vi "Init Tree.vi"(8 "error in":errorcluster) -> (0 "error out":errorcluster, 3 "Tree Map out":refnum<class "Project Tree Map.lvclass">)   [LabVIEW 2020, in "VI Properties Editor.lvlib" / "Project Tree Map.lvclass"]
doc: "Initializes the tree."
uses:
  Project Tree Map.lvclass
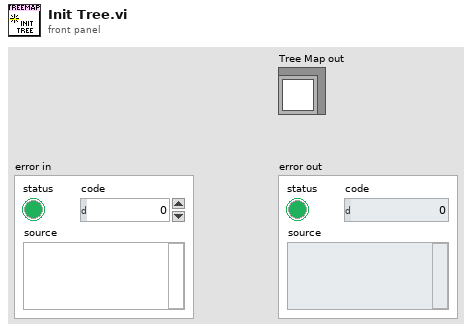
[diagram p1: front panel]
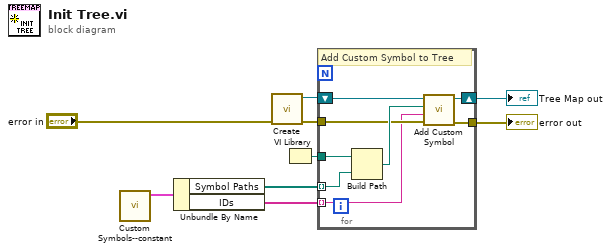
[diagram p0: block diagram]
diagram:
  n1 = call "Custom Symbols--constant.vi"() -> ("Custom Symbols"=w4:cluster{"Symbol Paths":path[], "IDs":string[]})  [unwired: 11 in]
  n2 = Unbundle By Name(w4) -> ("Symbol Paths"=w3:path[], "IDs"=w2:string[])
  n3 = call "Create.vi"("error in (no error)"="error in") -> ("error out"=w5:errorcluster, "Tree Map out"=w1:refnum<class "Project Tree Map.lvclass">)  [unwired: 9 in]
  n4 = VI Library() -> (path=w9:path)
  n5 = for {
    tunnel: w9 -> [w17]
    shift-right: [w14] -> w6
    shift-left: w1 -> [w16]
    tunnel: w5 -> [w12]
    tunnel: [w13] -> w8
    tunnel: w2 -> [w10] mode=indexing
    tunnel: w3 -> [w11] mode=indexing
    # "Add Custom Symbol to Tree"
    n6 = Build Path(base path=w17, name or relative path=w11) -> (appended path=w15:path)
    n7 = call "Add Custom Symbol.vi"("error in"=w12, "Symbol ID"=w10, "Symbol File Path"=w15, "Tree Map"=w16) -> ("error out"=w13:errorcluster, "Tree Map"=w14:refnum<class "Project Tree Map.lvclass">)  [unwired: 6 in]
  }
  "error out" <- w8
  "Tree Map out" <- w6
